vi "define_squarewave.vi"(1 "input cluster":T1={"base directory"=path "C:/Users/training/Desktop/Data", "data directory"=path "", "active"=FALSE, "running"=FALSE, "pairing"=FALSE, "clean tubes"=FALSE, "animal ID"=4, "session ID"=0, "base temp"=32.0, "d wait min"=500, "d wait max"=500, "d timeout"=5000, "d reward"=100, "idx stim"=0, "timeout win"=5000, "lick win"=[0, 100], "stim type"=[enum."pulse", enum."pulse", enum."pulse"], "stim dur"=[500, 400, 300], "stim amp"=[1.0, -1.0, 1.0], "stim freq"=[50, 50, 50], "stim ramp"=[1, 1, 1], "stim catch"=[0, 0, 1], "square dur"=[50, 20, 10], "square delay"=[50, 20, 10], "square freq"=[50, 50, 50], "square dc"=[50, 20, 10], "stim shape"=array3x500[1500 elements], "square shape"=[]} {"stim ramp" min=1}, 3 "error in":errorcluster) -> (8 "output cluster":T1={"base directory"=path "C:/Users/training/Desktop/Data", "data directory"=path "", "active"=FALSE, "running"=FALSE, "pairing"=FALSE, "clean tubes"=FALSE, "animal ID"=4, "session ID"=0, "base temp"=32.0, "d wait min"=500, "d wait max"=500, "d timeout"=5000, "d reward"=100, "idx stim"=0, "timeout win"=5000, "lick win"=[0, 100], "stim type"=[enum."pulse", enum."pulse", enum."pulse"], "stim dur"=[500, 400, 300], "stim amp"=[1.0, -1.0, 1.0], "stim freq"=[50, 50, 50], "stim ramp"=[1, 1, 1], "stim catch"=[0, 0, 1], "square dur"=[50, 20, 10], "square delay"=[50, 20, 10], "square freq"=[50, 50, 50], "square dc"=[50, 20, 10], "stim shape"=array3x500[1500 elements], "square shape"=[[TRUE, TRUE, TRUE, TRUE, TRUE, TRUE, TRUE, TRUE, TRUE, TRUE, FALSE, FALSE, FALSE, FALSE, FALSE, FALSE, FALSE, FALSE, FALSE, FALSE, TRUE, TRUE, TRUE, TRUE, TRUE, TRUE, TRUE, TRUE, TRUE, TRUE, FALSE, FALSE, FALSE, FALSE, FALSE, FALSE, FALSE, FALSE, FALSE, FALSE, TRUE, TRUE, TRUE, TRUE, TRUE, TRUE, TRUE, TRUE, TRUE, TRUE], [TRUE, TRUE, TRUE, TRUE, FALSE, FALSE, FALSE, FALSE, FALSE, FALSE, FALSE, FALSE, FALSE, FALSE, FALSE, FALSE, FALSE, FALSE, FALSE, FALSE, FALSE, FALSE, FALSE, FALSE, FALSE, FALSE, FALSE, FALSE, FALSE, FALSE, FALSE, FALSE, FALSE, FALSE, FALSE, FALSE, FALSE, FALSE, FALSE, FALSE, FALSE, FALSE, FALSE, FALSE, FALSE, FALSE, FALSE, FALSE, FALSE, FALSE], [TRUE, TRUE, FALSE, FALSE, FALSE, FALSE, FALSE, FALSE, FALSE, FALSE, FALSE, FALSE, FALSE, FALSE, FALSE, FALSE, FALSE, FALSE, FALSE, FALSE, FALSE, FALSE, FALSE, FALSE, FALSE, FALSE, FALSE, FALSE, FALSE, FALSE, FALSE, FALSE, FALSE, FALSE, FALSE, FALSE, FALSE, FALSE, FALSE, FALSE, FALSE, FALSE, FALSE, FALSE, FALSE, FALSE, FALSE, FALSE, FALSE, FALSE]]} {"stim ramp" min=1}, 10 "error out":errorcluster)   [LabVIEW 2016]
uses:
  Type Definitions/vars_settings.ctl
  Type Definitions/stim_type.ctl
  <vilib>/Analysis/NI_AALBase.lvlib
panel:
  out "squarewave":i16[][](graph)=[[1, 1, 1, 1, 1, 1, 1, 1, 1, 1, 0, 0, 0, 0, 0, 0, 0, 0, 0, 0, 1, 1, 1, 1, 1, 1, 1, 1, 1, 1, 0, 0, 0, 0, 0, 0, 0, 0, 0, 0, 1, 1, 1, 1, 1, 1, 1, 1, 1, 1], [1, 1, 1, 1, 0, 0, 0, 0, 0, 0, 0, 0, 0, 0, 0, 0, 0, 0, 0, 0, 0, 0, 0, 0, 0, 0, 0, 0, 0, 0, 0, 0, 0, 0, 0, 0, 0, 0, 0, 0, 0, 0, 0, 0, 0, 0, 0, 0, 0, 0], [1, 1, 0, 0, 0, 0, 0, 0, 0, 0, 0, 0, 0, 0, 0, 0, 0, 0, 0, 0, 0, 0, 0, 0, 0, 0, 0, 0, 0, 0, 0, 0, 0, 0, 0, 0, 0, 0, 0, 0, 0, 0, 0, 0, 0, 0, 0, 0, 0, 0]]
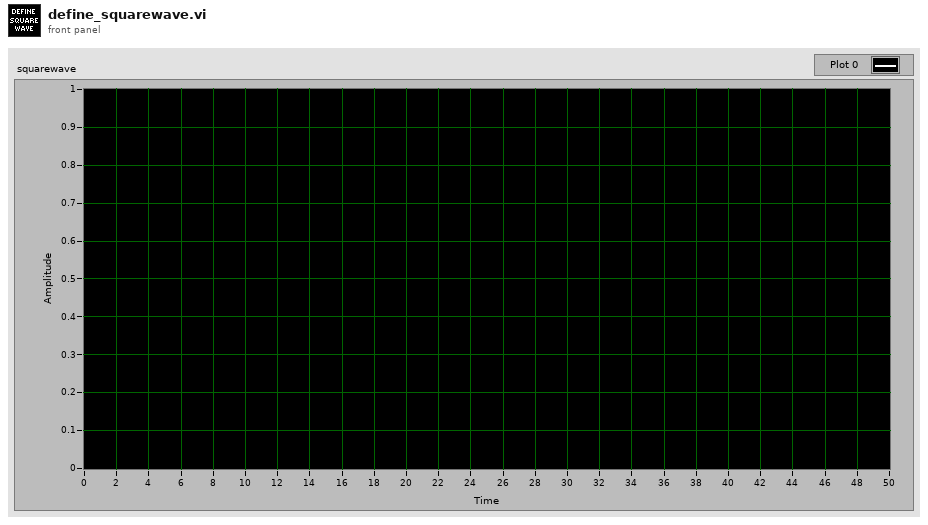
[diagram p1: front panel]
types:
  T1 = typedef "vars_settings.ctl" = cluster{"base directory":path, "data directory":path, "active":bool, "running":bool, "pairing":bool, "clean tubes":bool, "animal ID":u16, "session ID":u16, "base temp":dbl, "d wait min":u16, "d wait max":u16, "d timeout":u16, "d reward":u16, "idx stim":u16, "timeout win":u16, "lick win":i32[], "stim type":T2[], "stim dur":u16[], "stim amp":dbl[], "stim freq":u16[], "stim ramp":u16[], "stim catch":u8[], "square dur":u8[], "square delay":u8[], "square freq":u8[], "square dc":u8[], "stim shape":dbl[][], "square shape":bool[][]}
  T2 = typedef "stim_type.ctl" = enum16{"pulse", "vibration", "square", "sine"}
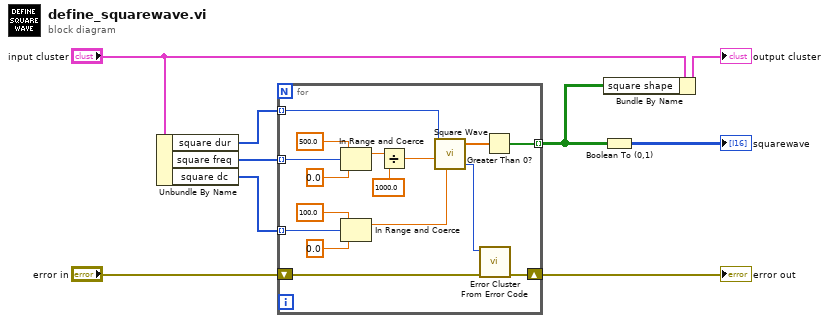
[diagram p0: block diagram]
diagram:
  n1 = Unbundle By Name("input cluster") -> ("square dur"=w7:u8[], "square freq"=w6:u8[], "square dc"=w5:u8[])
  n2 = for {
    tunnel: w6 -> [w16] mode=indexing
    tunnel: w5 -> [w15] mode=indexing
    tunnel: w7 -> [w14] mode=indexing
    shift-right: [w12] -> w1
    shift-left: "error in" -> [w11]
    tunnel: [w10] -> w2 mode=indexing
    n3 = In Range and Coerce(upper limit=500.0, x=w16, lower limit=0.0 ("upper limit")) -> (coerced(x)=w21:dbl)  [unwired: 1 out]
    n4 = In Range and Coerce(upper limit=100.0, x=w15, lower limit=0.0) -> (coerced(x)=w19:dbl)  [unwired: 1 out]
    n5 = Divide(x=w21, y=1000.0) -> (x/y=w17:dbl)
    n6 = call <vilib>:"Square Wave.vi"("samples"=w14, "frequency"=w17, "duty cycle (%)"=w19) -> ("square wave"=w25:dbl[], "error"=w13:i32)  [unwired: 3 in, 1 out]
    n7 = call <vilib>:"Error Cluster From Error Code.vi"("error in (no error)"=w11, "error code (0)"=w13) -> ("error out"=w12:errorcluster)  [unwired: 7 in]
    n8 = Greater Than 0?(x=w25) -> (x > 0?=w10:bool[])
  }
  "error out" <- w1
  n9 = Bundle By Name(cluster="input cluster", "square shape"=w2) -> (→"output cluster":T1)
  n10 = Boolean To (0,1)(Boolean=w2) -> (0, 1=→"squarewave":i16[][])
